vi "Initialize.vi"(7 "Process ID":string, 8 "error in (no error)":errorcluster, 10 "Device Item Ref":T1=18446744073709551615 format="%.0x", 11 "Process in":refnum<class "Process.lvclass">) -> (0 "error out":errorcluster, 3 "Process out":refnum<class "Process.lvclass">)   [LabVIEW 2019, in "TimingDRV Engine.lvlib" / "Process.lvclass"]
uses:
  Process.lvclass
  <vilib>/NI VeriStand/Custom Device API/Custom Device Item Ref.ctl
  TypeDefs/Message.ctl
  TypeDefs/Update.ctl
  Process.lvclass/Process.ctl
  <vilib>/NI VeriStand/Custom Device API/Custom Device API.lvlib
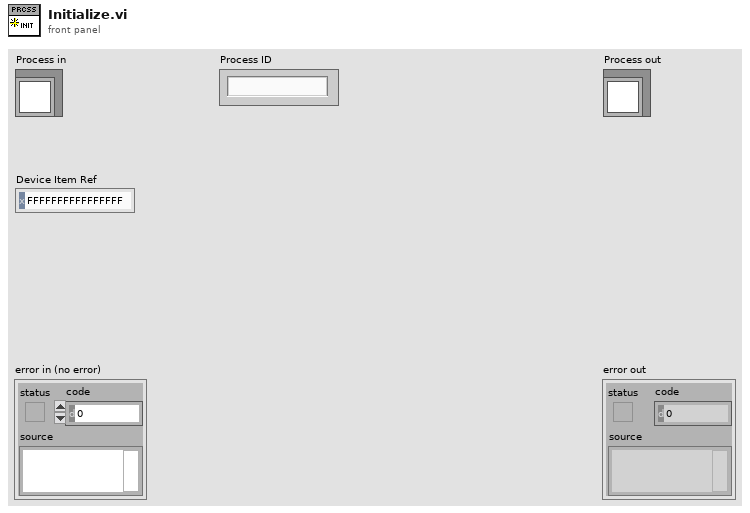
[diagram p1: front panel]
types:
  T1 = typedef "Custom Device API.lvlib/Custom Device Item Ref.ctl" = u64
  T2 = typedef "TimingDRV Engine.lvlib/Process.lvclass/Update.ctl" = cluster{"Update Message":string, "Payload":variant}
  T3 = typedef "TimingDRV Engine.lvlib/Process.lvclass/Message.ctl" = cluster{"Command":string, "Payload":variant}
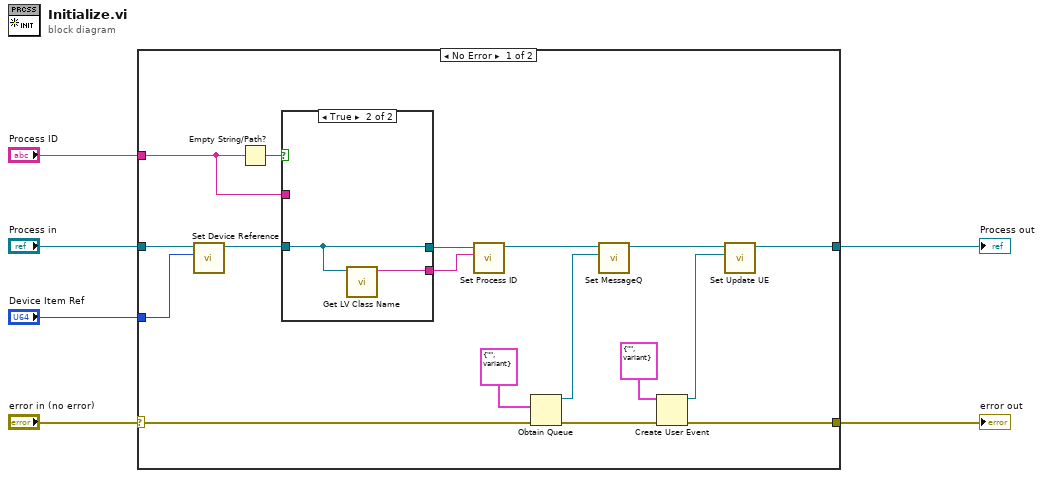
[diagram p0: block diagram]
diagram:
  n1 = case shown="No Error" "error in (no error)" {
    selector: "error in (no error)" -> [w23 w29]
    tunnel: [w15 w29] -> w5
    tunnel: [w7 w28] -> w3
    tunnel: "Process in" -> [w14 w28]
    tunnel: "Process ID" -> [w11 _]
    tunnel: "Device Item Ref" -> [w13 _]
    frame No Error {
      n2 = call "Set Device Reference.vi"("Device Item Ref"=w13, "CD_Process in"=w14) -> ("CD_Process out"=w10:refnum<class "Process.lvclass">)  [unwired: 9 in]
      n3 = Empty String/Path?(string/path=w11) -> (empty?=w12:bool)
      n4 = case shown="True" w12 {
        tunnel: w11 -> [w25 _]
        tunnel: w10 -> [w24 w27]
        tunnel: [w24 w27] -> w9
        tunnel: [w25 w26] -> w8
        frame False {
        }
        frame True {
          n5 = call <vilib>:"Get LV Class Name.vi"("object"=w27) -> ("class name"=w26:string)  [unwired: 9 in, 1 out]
        }
      }
      n6 = call "Set Process ID.vi"("Process ID"=w8, "CD_Process in"=w9) -> ("CD_Process out"=w20:refnum<class "Process.lvclass">)  [unwired: 9 in]
      n7 = Obtain Queue(element data type=T3 {"Command"="", "Payload"=variant}, error in (no error)=w23) -> (queue out=w21:refnum<queue>, error out=w19:errorcluster)  [unwired: 3 in, 1 out]
      n8 = call "Set MessageQ.vi"("MessageQ"=w21, "CD_Process in"=w20) -> ("CD_Process out"=w17:refnum<class "Process.lvclass">)  [unwired: 9 in]
      n9 = Create User Event(user event datatype=T2 {"Update Message"="", "Payload"=variant} ("Update"), error in=w19) -> (user event=w16:refnum<user-event>, error out=w15:errorcluster)
      n10 = call "Set Update UE.vi"("Update UE"=w16, "CD_Process in"=w17) -> ("CD_Process out"=w7:refnum<class "Process.lvclass">)  [unwired: 9 in]
    }
    frame Error {
    }
  }
  "error out" <- w5
  "Process out" <- w3
